vi "EPICS_VALVE_HANDLE.vi"(9 "OPEN_Vn_REQ_IN":bool, 10 "Vn_CLOSE":bool, 11 "n_OPEN":bool) -> (3 "OPEN_Vn_REQ_OUT":bool)   [LabVIEW 2015]
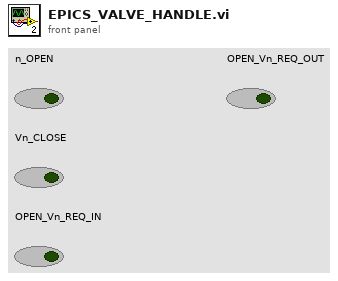
[diagram p1: front panel]
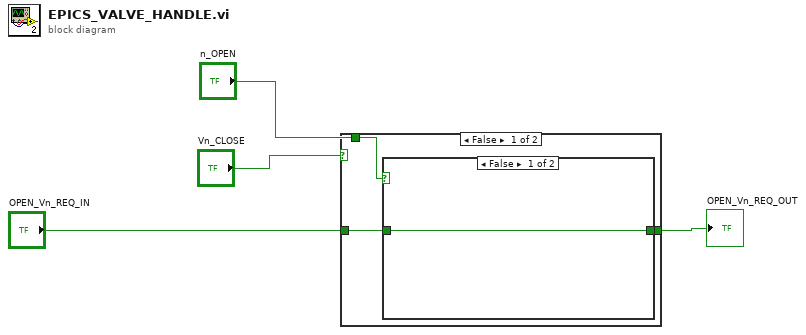
[diagram p0: block diagram]
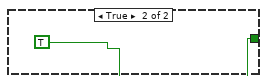
[diagram p2: hidden frame]
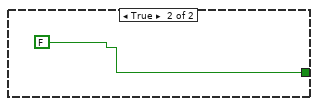
[diagram p3: hidden frame]
diagram:
  n1 = case shown="False" "Vn_CLOSE" {
    tunnel: [w6 FALSE ("APX:V4_OPEN_REQ")] -> w2
    tunnel: "n_OPEN" -> [w7 _]
    tunnel: "OPEN_Vn_REQ_IN" -> [w5 _]
    frame False {
      n2 = case shown="False" w7 {
        tunnel: [w8 TRUE ("APX:V4_OPEN_REQ")] -> w6
        tunnel: w5 -> [w8 _]
        frame False {
        }
        frame True {
        }
      }
    }
    frame True {
    }
  }
  "OPEN_Vn_REQ_OUT" <- w2
